vi "ExpDestroyMatlabEnv.vi"(8 "error in (no error)":errorcluster) -> (0 "error out":errorcluster)   [LabVIEW 2017]
uses:
  ExpGlobals.vi
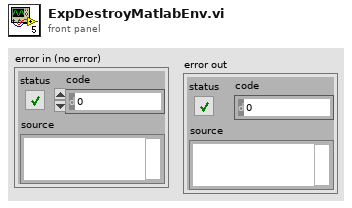
[diagram p1: front panel]
types:
  T1 = enum32{"Invalid", "Standard", "Closed", "Hidden", "Minimized", "Maximized"}
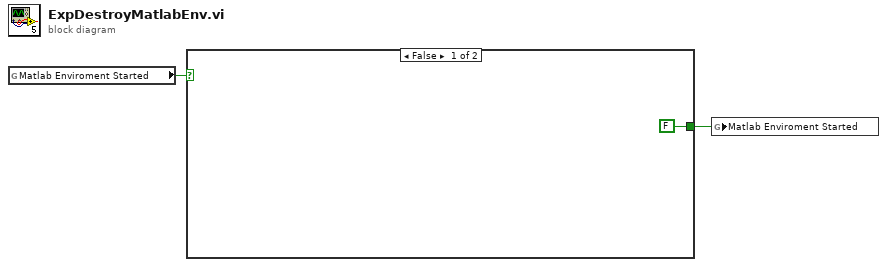
[diagram p0: block diagram]
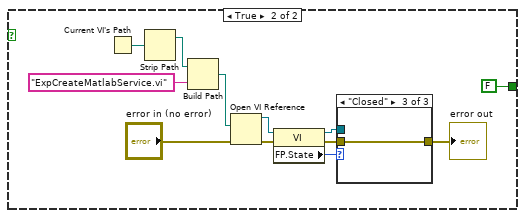
[diagram p2: hidden frame]
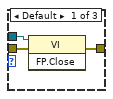
[diagram p3: hidden frame]
diagram:
  n1 = global read "ExpGlobals.vi" "Matlab Enviroment Started"() -> (w2:bool)
  n2 = case shown="False" w2 {
    tunnel: [FALSE FALSE] -> w1
    frame False {
    }
    frame True {
      n3 = Current VI's Path() -> (path=w12:path)
      n4 = Strip Path(path=w12) -> (stripped path=w11:path)  [unwired: 1 out]
      n5 = Build Path(base path=w11, name or relative path="ExpCreateMatlabService.vi") -> (appended path=w10:path)
      n6 = Open VI Reference(vi path=w10, error in (no error)="error in (no error)") -> (vi reference=w9:refnum<vi>, error out=w7:errorcluster)  [unwired: 4 in]
      n7 = property class="VI"(reference=w9, error in=w7) -> (reference out=w8:refnum<vi>, error out=w6:errorcluster, "FP.State"=w5:T1)
      n8 = case shown="\"Closed\"" w5 {
        tunnel: [w18 w19 w20] -> w15
        tunnel: w8 -> [w17 _ _]
        tunnel: w6 -> [w16 w19 w20]
        frame Default {
          n9 = invoke class="VI" method="FP.Close"(reference=w17, error in=w16) -> (error out=w18:errorcluster)  [unwired: 1 in, 2 out]
        }
        frame "Invalid" {
        }
        frame "Closed" {
        }
      }
      "error out" <- w15
    }
  }
  n10 = global write "ExpGlobals.vi" "Matlab Enviroment Started"(w1) -> ()
